vi "EventQueueCreate.vi"(2 "error in (no error)":errorcluster) -> (0 "EventError":errorcluster, 1 "EventQueue":refnum<queue>)   [LabVIEW 2017]
uses:
  EventQueueCluster.ctl
  EventMessage.ctl
panel:
  in  "String":string
  in  "EventQueueCluster":T1={"EventsMessage"=enum."Init", "NumericValue"=0.0, "String"=""}
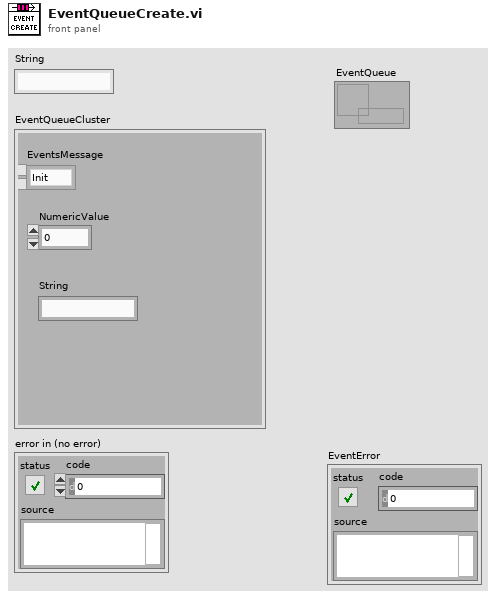
[diagram p1: front panel]
types:
  T1 = typedef "EventQueueCluster.ctl" = cluster{"EventsMessage":T2, "NumericValue":dbl, "String":string}
  T2 = typedef "EventMessage.ctl" = enum16{"Error", "Init", "Listen", "Halt"}
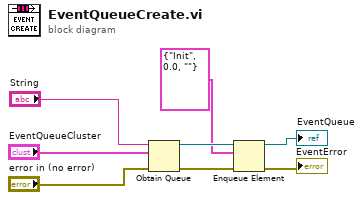
[diagram p0: block diagram]
diagram:
  n1 = Obtain Queue(name (unnamed)="String", element data type="EventQueueCluster", error in (no error)="error in (no error)") -> (queue out=w6:refnum<queue>, error out=w5:errorcluster)  [unwired: 2 in, 1 out]
  n2 = Enqueue Element(queue=w6, element=T1 {"EventsMessage"=enum."Init", "NumericValue"=0.0, "String"=""}, error in (no error)=w5) -> (queue out=→"EventQueue":refnum<queue>, error out=→"EventError":errorcluster)  [unwired: 1 in, 1 out]
